vi "Write Element of Image.vi"(9 "Image":T1, 10 "index":i32, 11 "CCD in":refnum<class "CCD.lvclass">) -> (3 "CCD out":refnum<class "CCD.lvclass">)   [LabVIEW 2016, in "Hardware.lvlib" / "CCD.lvlib" / "CCD.lvclass"]
uses:
  <userlib>/Common Components/Hardware/CCD/CCD/CCD.lvclass
  <vilib>/vision/Image Controls.llb/IMAQ Image.ctl
  <userlib>/Common Components/Hardware/CCD/CCD/CCD.lvclass/CCD.ctl
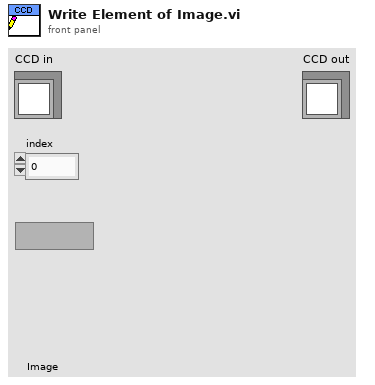
[diagram p1: front panel]
types:
  T1 = typedef "IMAQ Image.ctl" = refnum<image>
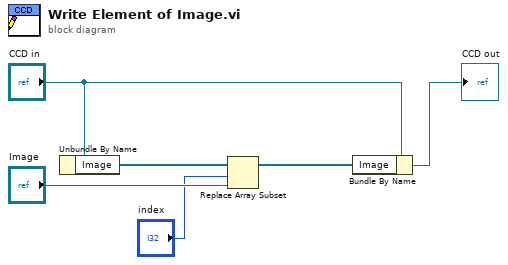
[diagram p0: block diagram]
diagram:
  n1 = Unbundle By Name("CCD in") -> ("Image"=w3:T1[])
  n2 = Replace Array Subset(array=w3, new element="Image", index="index") -> (w2:T1[])
  n3 = Bundle By Name(cluster="CCD in", "Image"=w2) -> (→"CCD out":refnum<class "CCD.lvclass">)
